vi "Automat_Lift_sbRIO.vi"() -> ()   [LabVIEW 2014]
uses:
  Timer/Timer/Control Timer.ctl
panel:
  out "Trenutno stanje":enum16{"Idle", "Moving", "DoorOpen", "Shutdown"}(ring)
  out "Grafik":dbl(graph)
  out "u":dbl
  out "x":dbl
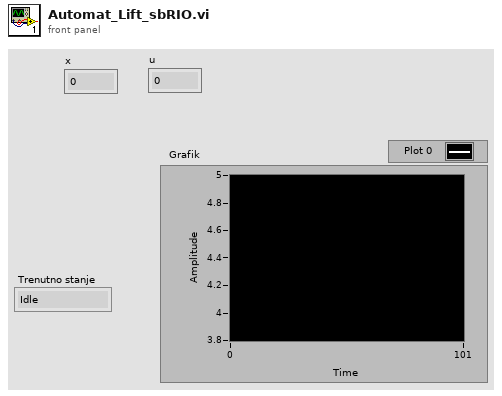
[diagram p1: front panel]
types:
  T1 = typedef "Control Timer.ctl" = enum16{"Timecheck", "Reset"}
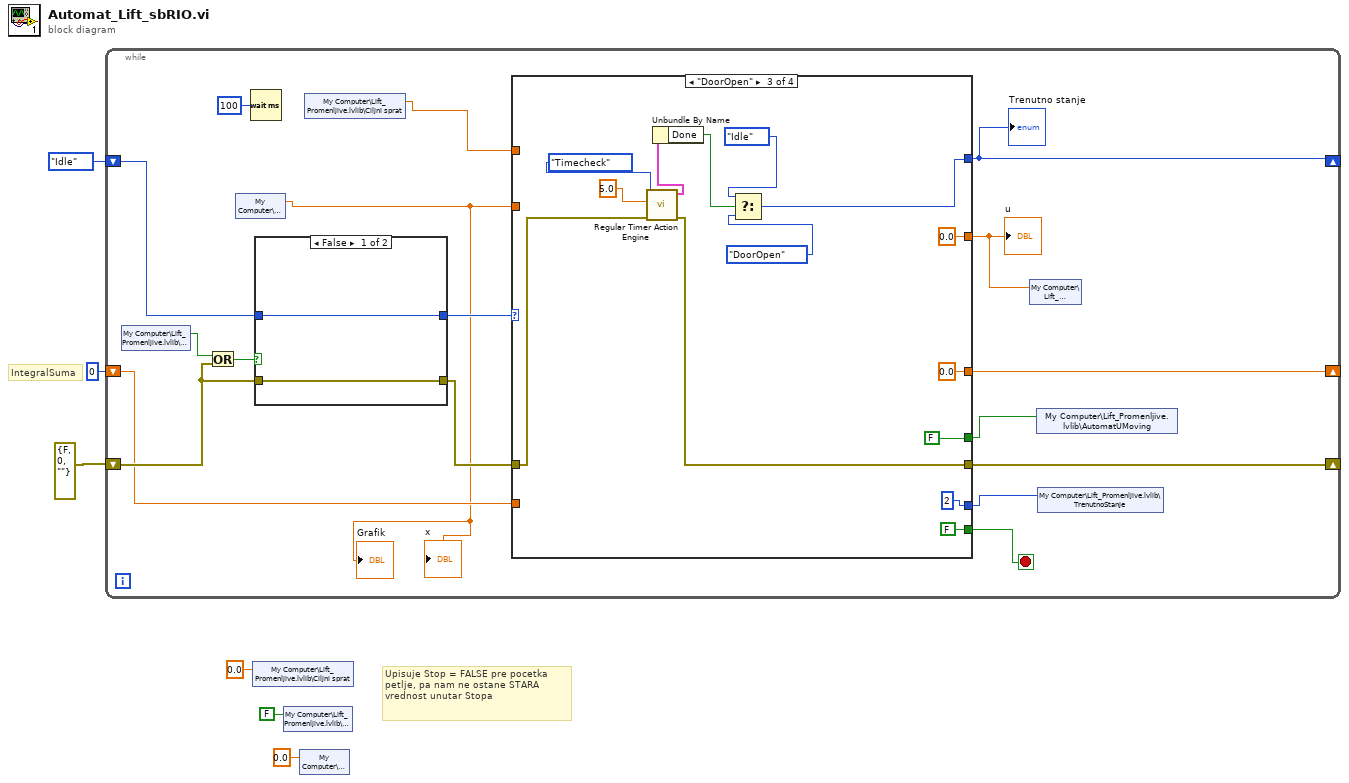
[diagram p0: block diagram]
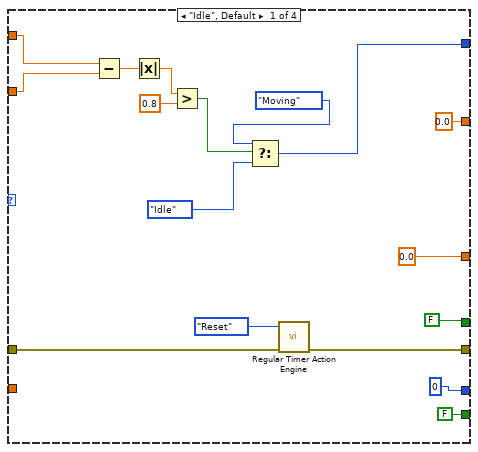
[diagram p2: hidden frame]
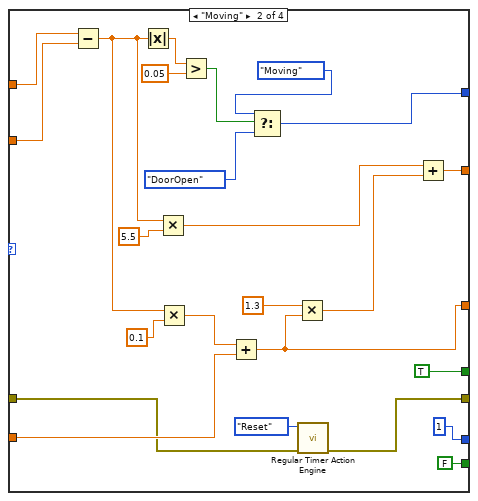
[diagram p3: hidden frame]
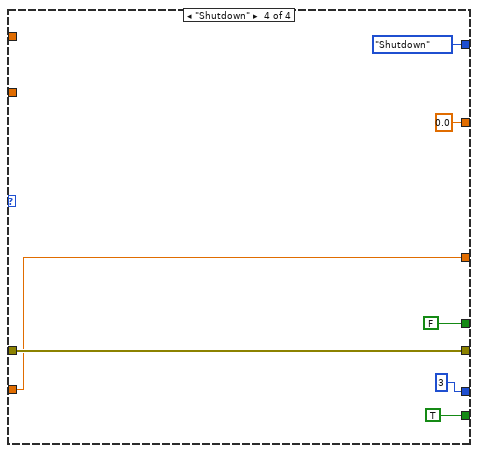
[diagram p4: hidden frame]
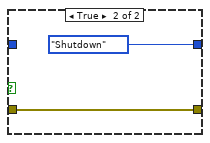
[diagram p5: hidden frame]
diagram:
  # "Upisuje Stop = FALSE pre pocetka petlje, pa nam ne ostane STARA vrednost unutar Stopa"
  # "IntegralSuma"
  n1 = while {
    shift-right: [w16] -> _
    shift-left: enum16{"Idle", "Moving", "DoorOpen", "Shutdown"}."Idle" ("Stanja") -> [w22]
    shift-right: [w19] -> _
    shift-left: 0 -> [w13]
    shift-right: [w21] -> _
    shift-left: errorcluster {"status"=FALSE, "code"=0, "source"=""} ("error constant") -> [w14]
    stop <- w18 stop-if-true
    n2 = shared-variable "My Computer\\Lift_Promenljive.lvlib\\Stop"() -> (w12:bool)  [unwired: 1 in, 1 out]
    n3 = Or(x=w12, y=w14) -> (x .or. y?=w23:bool)
    n4 = shared-variable "My Computer\\Lift_Promenljive.lvlib\\x"() -> (w11:dbl)  [unwired: 1 in, 1 out]
    "x" <- w11
    "Grafik" <- w11
    n5 = Wait (ms)(milliseconds to wait=u32 100) -> ()  [unwired: 1 out]
    n6 = case shown="False" w23 {
      tunnel: [w87 enum16{"Idle", "Moving", "DoorOpen", "Shutdown"}."Shutdown" ("Stanja")] -> w15
      tunnel: w22 -> [w87 _]
      tunnel: w14 -> [w86 w88]
      tunnel: [w86 w88] -> w20
      frame False {
      }
      frame True {
      }
    }
    n7 = shared-variable "My Computer\\Lift_Promenljive.lvlib\\Ciljni sprat"() -> (w10:dbl)  [unwired: 1 in, 1 out]
    n8 = case shown="\"DoorOpen\"" w15 {
      tunnel: w11 -> [w26 w59 _ _]
      tunnel: w13 -> [_ w52 _ w82]
      tunnel: w10 -> [w36 w56 _ _]
      tunnel: [w35 w60 w76 enum16{"Idle", "Moving", "DoorOpen", "Shutdown"}."Shutdown" ("Stanja")] -> w16
      tunnel: [w28 w47 w72 w83] -> w21
      tunnel: w20 -> [w27 w46 w73 w83]
      tunnel: [0.0 w51 0.0 w82] -> w19
      tunnel: [0.0 w44 0.0 0.0] -> w9
      tunnel: [FALSE FALSE FALSE TRUE] -> w18
      tunnel: [FALSE TRUE FALSE FALSE] -> w8
      tunnel: [0 1 2 3] -> w7
      frame "Idle", Default {
        n9 = Subtract(x=w36, y=w26) -> (x-y=w31:dbl)
        n10 = Absolute Value(x=w31) -> (abs(x)=w30:dbl)
        n11 = Greater?(x=w30, y=0.8) -> (0:w39:bool)
        n12 = Select(t=enum16{"Idle", "Moving", "DoorOpen", "Shutdown"}."Moving" ("Stanja"), s=w39, f=enum16{"Idle", "Moving", "DoorOpen", "Shutdown"}."Idle" ("Stanja")) -> (s? t:f=w35:enum16{"Idle", "Moving", "DoorOpen", "Shutdown"})
        n13 = call "Regular Timer Action Engine.vi"("Enum"=Control_Timer."Reset", "error in"=w27) -> ("error out"=w28:errorcluster)  [unwired: 7 in, 1 out]
      }
      frame "Moving" {
        n14 = Subtract(x=w56, y=w59) -> (x-y=w55:dbl)
        n15 = Absolute Value(x=w55) -> (abs(x)=w48:dbl)
        n16 = Multiply(x=w55, y=5.5) -> (x*y=w49:dbl)
        n17 = Multiply(x=w55, y=0.1) -> (x*y=w53:dbl)
        n18 = Greater?(x=w48, y=0.05) -> (0:w63:bool)
        n19 = Add(x=w53, y=w52) -> (x+y=w51:dbl)
        n20 = Select(t=enum16{"Idle", "Moving", "DoorOpen", "Shutdown"}."Moving" ("Stanja"), s=w63, f=enum16{"Idle", "Moving", "DoorOpen", "Shutdown"}."DoorOpen" ("Stanja")) -> (s? t:f=w60:enum16{"Idle", "Moving", "DoorOpen", "Shutdown"})
        n21 = Multiply(x=1.3, y=w51) -> (x*y=w43:dbl)
        n22 = call "Regular Timer Action Engine.vi"("Enum"=Control_Timer."Reset", "error in"=w46) -> ("error out"=w47:errorcluster)  [unwired: 7 in, 1 out]
        n23 = Add(x=w49, y=w43) -> (x+y=w44:dbl)
      }
      frame "DoorOpen" {
        n24 = call "Regular Timer Action Engine.vi"("Enum"=Control_Timer."Timecheck", "Time Target"=5.0, "error in"=w73) -> ("Status"=w69:cluster{"Running":bool, "Done":bool}, "error out"=w72:errorcluster)  [unwired: 6 in]
        n25 = Unbundle By Name(w69) -> ("Done"=w68:bool)
        n26 = Select(t=enum16{"Idle", "Moving", "DoorOpen", "Shutdown"}."Idle" ("Stanja"), s=w68, f=enum16{"Idle", "Moving", "DoorOpen", "Shutdown"}."DoorOpen" ("Stanja")) -> (s? t:f=w76:enum16{"Idle", "Moving", "DoorOpen", "Shutdown"})
      }
      frame "Shutdown" {
      }
    }
    "u" <- w9
    "Trenutno stanje" <- w16
    n27 = shared-variable "My Computer\\Lift_Promenljive.lvlib\\u"(w9) -> ()  [unwired: 1 in, 1 out]
    n28 = shared-variable "My Computer\\Lift_Promenljive.lvlib\\AutomatUMoving"(w8) -> ()  [unwired: 1 in, 1 out]
    n29 = shared-variable "My Computer\\Lift_Promenljive.lvlib\\TrenutnoStanje"(w7) -> ()  [unwired: 1 in, 1 out]
  }
  n30 = shared-variable "My Computer\\Lift_Promenljive.lvlib\\Ciljni sprat"(0.0 ("Ciljni sprat")) -> ()  [unwired: 1 in, 1 out]
  n31 = shared-variable "My Computer\\Lift_Promenljive.lvlib\\Stop"(FALSE ("Stop")) -> ()  [unwired: 1 in, 1 out]
  n32 = shared-variable "My Computer\\Lift_Promenljive.lvlib\\x"(0.0 ("x")) -> ()  [unwired: 1 in, 1 out]
